vi "Framework.Set Debug Flags.vi"(10 "Debug Flags":refnum<class "Debug Flags.lvclass">, 11 "Framework in":refnum<class "Framework.lvclass">) -> (3 "Framework out":refnum<class "Framework.lvclass">)   [LabVIEW 2017, in "DSF Core.lvlib" / "Framework.lvclass"]
uses:
  Framework.lvclass
  Debug/Debug Flags/Debug Flags.lvclass
  Framework.lvclass/Framework.ctl
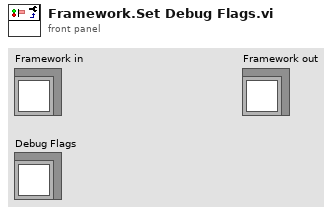
[diagram p1: front panel]
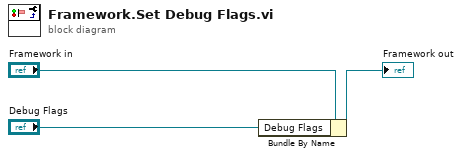
[diagram p0: block diagram]
diagram:
  n1 = Bundle By Name(cluster="Framework in", "Debug Flags"="Debug Flags") -> (→"Framework out":refnum<class "Framework.lvclass">)
